vi "Control Experiment.vi"() -> ()   [LabVIEW 2016, in "Transport.lvclass"]
uses:
  Transport.lvclass
  <userlib>/LevyLab/Krohn Hite 7008/SMOs/KH7008/typedefs/Shunt-Enum.ctl
  <userlib>/LevyLab/Krohn Hite 7008/SMOs/KH7008/typedefs/Gain-Enum.ctl
  <userlib>/LevyLab/Krohn Hite 7008/SMOs/KH7008/typedefs/KH_control_array.ctl
  <userlib>/LevyLab/Krohn Hite 7008/SMOs/KH7008/typedefs/KH_control.ctl
  <userlib>/LevyLab/Krohn Hite 7008/SMOs/KH7008/typedefs/Channel-Enum.ctl
  <userlib>/LevyLab/Krohn Hite 7008/SMOs/KH7008/typedefs/Input Configuration-Enum.ctl
  ITX_Global.vi
  <userlib>/LevyLab/Krohn Hite 7008/SMOs/KH7008/KH7008.lvclass
panel:
  in  "canvas":string="SA01234"
  out "filename":string="SA01234.20180713"
  out "folder":string="G:\\Team Drives\\LevyLabData/quasi-1D chiral proteins/SA01234.20180713"
  out "comments":string="SA01234.20180713\nquasi-1D chiral proteins\npatrick"
  in  "user (emum?)":string="patrick"
  in  "project (enum?)":string="quasi-1D chiral proteins"
  out "device":string="SA01234.20180713"
  in  "device":string="20180713"
  in  "sample":string="SA01234"
  in  "all grounded":bool
  in  "Label":T1(array[ring])
  in  "Lockin Ch":enum16{"1", "2", "3", "4", "5", "6", "7", "8"}[](array[ring])=[enum."1", enum."2", enum."3", enum."4", enum."5", enum."6", enum."7", enum."8"]
  in  "Electrode":T2(array[ring])
  in  "KH Ch":enum16{"1", "2", "3", "4", "5", "6", "7", "8"}[](array[ring])=[enum."1", enum."2", enum."3", enum."4", enum."5", enum."6", enum."7", enum."8"]
  in  "all shunt same":bool
  in  "all gain same":bool
  in  "All same as ch1?":bool
  in  "Gain":T3[](array[typedef])
  in  "Shunt Resistor":T4[](array[typedef])
  in  "Configuration":enum16{"Ground", "Current", "Voltage", "Gate"}[](array[ring])=[enum."Current"]
  # "some of these are used to set KH\nsome are just saved as meta data\nsome are used"
  # "how to sell?\nshow what it is replacing\n(KH control, Channel Globals, Lockin 0 vs 1 nonsene, typing into comments)"
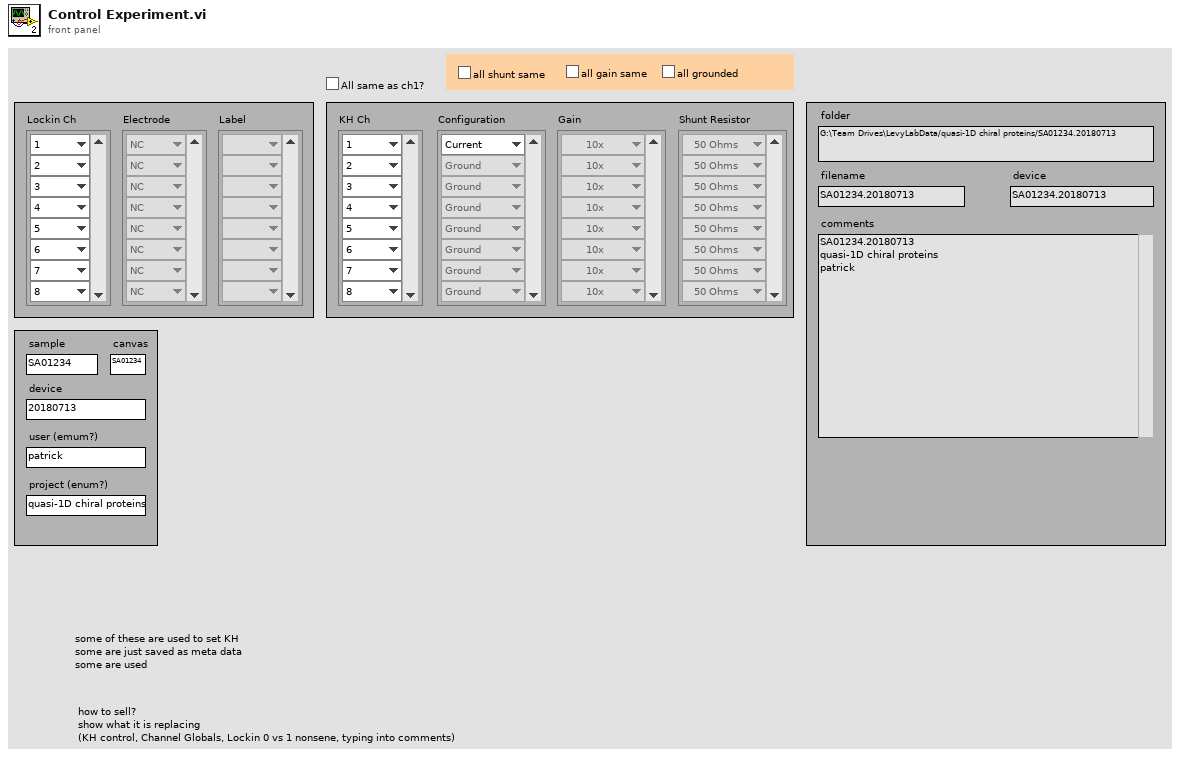
[diagram p1: front panel]
types:
  T1 = enum16{"", "I+", "I-", "V1+", "V1-", "V2+", "V2-", "V3+", "V3-", "Vsg1", "Vsg2", "Vsg3", "Vbg"}[]
  T2 = enum16{"NC", "26", "27", "28", "1", "2", "3", "4", "5", "6", "7", "8", "9", "10", "11", "12", "13", "14", "15", "16", "17", "18", "19", "20", "21", "22", "23", "24", "25"}[]
  T3 = typedef "KH7008.lvclass/Gain-Enum.ctl" = enum16{"1x", "10x", "100x", "1000x"}
  T4 = typedef "KH7008.lvclass/Shunt-Enum.ctl" = enum16{"Open", "50 Ohms", "500 Ohms", "5k Ohms", "50k Ohms"}
  T5 = typedef "KH7008.lvclass/KH_control_array.ctl" = T6[]
  T6 = typedef "KH7008.lvclass/KH_control.ctl" = cluster{"Channel":T7, "Gain":T3, "Shunt Resistor":T4, "Input Config":T8}
  T7 = typedef "KH7008.lvclass/Channel-Enum.ctl" = enum16{"Channel 1", "Channel 2", "Channel 3", "Channel 4", "Channel 5", "Channel 6", "Channel 7", "Channel 8"}
  T8 = typedef "KH7008.lvclass/Input Configuration-Enum.ctl" = enum16{"Ground", "SE+ (-gnd)", "SE- (+gnd)", "Differential"}
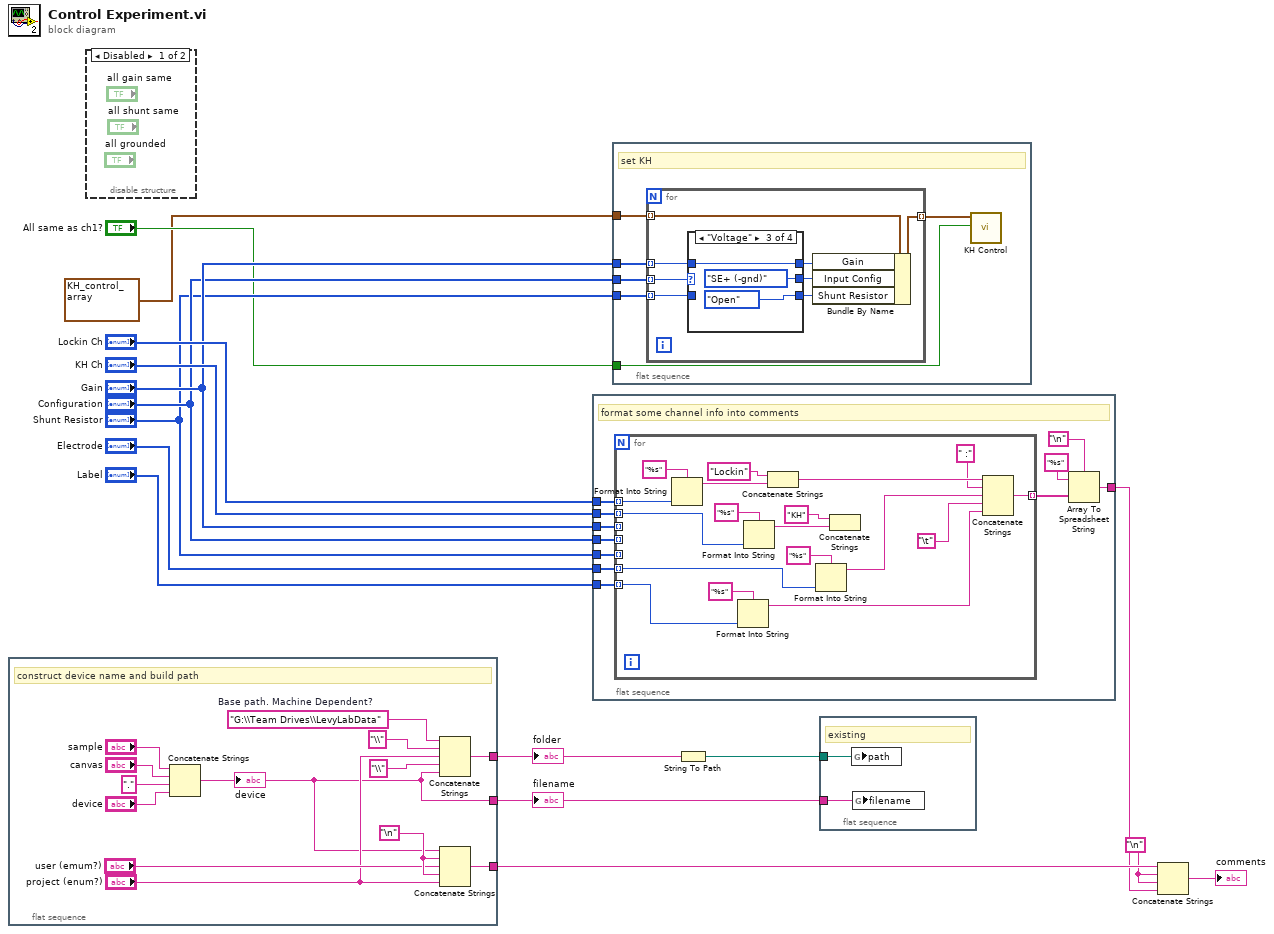
[diagram p0: block diagram]
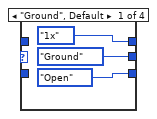
[diagram p2: hidden frame]
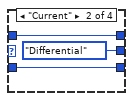
[diagram p3: hidden frame]
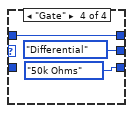
[diagram p4: hidden frame]
diagram:
  w8 = "\n"
  n1 = flat-sequence {
    tunnel: [w19] -> w9
    tunnel: [w18] -> w5
    tunnel: [w17] -> w4
    frame #0 {
      w22 = "\n"
      w28 = "G:\\Team Drives\\LevyLabData"  # Base path. Machine Dependent?
      # "construct device name and build path"
      n2 = Concatenate Strings("sample", "canvas", "." ("string"), "device") -> (w18:string)
      "device" <- w18
      n3 = Concatenate Strings(w28, "\\" ("string"), "project (enum?)", "\\" ("string"), w18) -> (w17:string)
      n4 = Concatenate Strings(w18, w22, "user (emum?)", w22, "project (enum?)") -> (w19:string)
    }
  }
  n5 = disable-structure shown="Disabled" {
    frame Disabled {
    }
    frame Enabled {
    }
  }
  n6 = flat-sequence {
    tunnel: "Lockin Ch" -> [w40]
    tunnel: "KH Ch" -> [w39]
    tunnel: "Gain" -> [w38]
    tunnel: "Configuration" -> [w37]
    tunnel: "Shunt Resistor" -> [w36]
    tunnel: "Electrode" -> [w35]
    tunnel: "Label" -> [w34]
    tunnel: [w30] -> w6
    frame #0 {
      # "format some channel info into comments"
      n7 = for {
        tunnel: w40 -> [w58] mode=indexing
        tunnel: w39 -> [w50] mode=indexing
        tunnel: w38 -> [_] mode=indexing
        tunnel: w37 -> [_] mode=indexing
        tunnel: w36 -> [_] mode=indexing
        tunnel: w35 -> [w41] mode=indexing
        tunnel: w34 -> [w49] mode=indexing
        tunnel: [w47] -> w33 mode=indexing
        n8 = Format Into String(format string="%s", w58) -> (resulting string=w55:string)  [unwired: 2 in, 1 out]
        n9 = Format Into String(format string="%s", w49) -> (resulting string=w43:string)  [unwired: 2 in, 1 out]
        n10 = Format Into String(format string="%s", w50) -> (resulting string=w54:string)  [unwired: 2 in, 1 out]
        n11 = Concatenate Strings("Lockin", w55) -> (w51:string)
        n12 = Format Into String(format string="%s", w41) -> (resulting string=w44:string)  [unwired: 2 in, 1 out]
        n13 = Concatenate Strings("KH", w54) -> ()  [unwired: 1 out]
        n14 = Concatenate Strings(w51, " :", w44, "\t", w43) -> (w47:string)
      }
      n15 = Array To Spreadsheet String(delimiter (Tab)="\n", array=w33, 3:"%s" ("format string")) -> (spreadsheet string=w30:string)
    }
  }
  n16 = flat-sequence {
    tunnel: "Gain" -> [w63]
    tunnel: "Configuration" -> [w62]
    tunnel: "Shunt Resistor" -> [w61]
    tunnel: "All same as ch1?" -> [w59]
    tunnel: T5 [{"Channel"=enum."Channel 1", "Gain"=enum."1x", "Shunt Resistor"=enum."Open", "Input Config"=enum."Ground"}, {"Channel"=enum."Channel 2", "Gain"=enum."1x", "Shunt Resistor"=enum."Open", "Input Config"=enum."Ground"}, {"Channel"=enum."Channel 3", "Gain"=enum."1x", "Shunt Resistor"=enum."Open", "Input Config"=enum."Ground"}, {"Channel"=enum."Channel 4", "Gain"=enum."1x", "Shunt Resistor"=enum."Open", "Input Config"=enum."Ground"}, {"Channel"=enum."Channel 5", "Gain"=enum."1x", "Shunt Resistor"=enum."Open", "Input Config"=enum."Ground"}, {"Channel"=enum."Channel 6", "Gain"=enum."1x", "Shunt Resistor"=enum."Open", "Input Config"=enum."Ground"}, {"Channel"=enum."Channel 7", "Gain"=enum."1x", "Shunt Resistor"=enum."Open", "Input Config"=enum."Ground"}, {"Channel"=enum."Channel 8", "Gain"=enum."1x", "Shunt Resistor"=enum."Open", "Input Config"=enum."Ground"}] ("Channel Setting") -> [w60]
    frame #0 {
      # "set KH"
      n17 = for {
        tunnel: w60 -> [w71] mode=indexing
        tunnel: w62 -> [w72] mode=indexing
        tunnel: [w69] -> w64 mode=indexing
        tunnel: w63 -> [w67] mode=indexing
        tunnel: w61 -> [w65] mode=indexing
        n18 = case shown="\"Voltage\"" w72 {
          tunnel: [Input_Configuration-Enum."Ground" ("Input Config") Input_Configuration-Enum."Differential" ("Input Config") Input_Configuration-Enum."SE+ (-gnd)" ("Input Config") Input_Configuration-Enum."Differential" ("Input Config")] -> w70
          tunnel: [Shunt-Enum."Open" ("Shunt Resistor") w76 Shunt-Enum."Open" ("Shunt Resistor") Shunt-Enum."50k Ohms" ("Shunt Resistor")] -> w68
          tunnel: w67 -> [_ w77 w80 w83]
          tunnel: [Gain-Enum."1x" ("Gain") w77 w80 w83] -> w66
          tunnel: w65 -> [_ w76 _ _]
          frame "Ground", Default {
          }
          frame "Current" {
          }
          frame "Voltage" {
          }
          frame "Gate" {
          }
        }
        n19 = Bundle By Name(cluster=w71, "Gain"=w66, "Input Config"=w70, "Shunt Resistor"=w68) -> (w69:T6)
      }
      n20 = call <userlib>:"KH Control.vi"("All same as ch1?"=w59, "Channel Setting"=w64) -> ()  [unwired: 8 in, 2 out]
    }
  }
  n21 = String To Path(string=w4) -> (path=w3:path)
  n22 = flat-sequence {
    tunnel: w5 -> [w86]
    tunnel: w3 -> [w85]
    frame #0 {
      # "existing"
      n23 = global write "ITX_Global.vi" "path"(w85) -> ()
      n24 = global write "ITX_Global.vi" "filename"(w86) -> ()
    }
  }
  n25 = Concatenate Strings(w9, w8, w8, w6) -> (→"comments":string)
  "folder" <- w4
  "filename" <- w5
